vi "Get Min Meter ROI.vi"(8 "error in (no error)":errorcluster, 11 "Item Ref in":T2 format="%.0x") -> (0 "error out":errorcluster, 1 "empty?":bool, 2 "Max Gauge ROI":T1, 3 "Item Ref out":T2 format="%.0x")   [LabVIEW 2011, in "Meter Detection Custom Device.lvlib"]
uses:
  Meter Detection Custom Device.lvlib
  <vilib>/NI Veristand/Custom Device API/Custom Device Item Ref.ctl
  Meter Detection Global Variable.vi
  <vilib>/NI Veristand/Custom Device API/Get Item Property (Variant).vi
  <vilib>/NI Veristand/Custom Device API/Custom Device API.lvlib
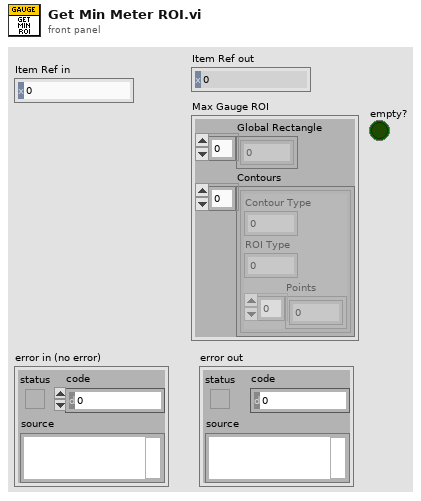
[diagram p1: front panel]
types:
  T1 = cluster{"Global Rectangle":i32[], "Contours":cluster{"Contour Type":u32, "ROI Type":u32, "Points":i32[]}[]}
  T2 = typedef "Custom Device API.lvlib/Custom Device Item Ref.ctl" = u64
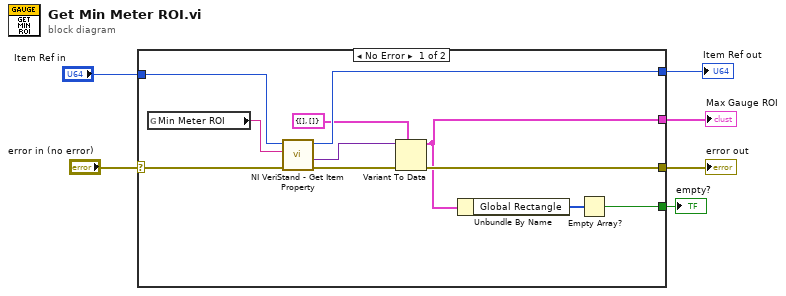
[diagram p0: block diagram]
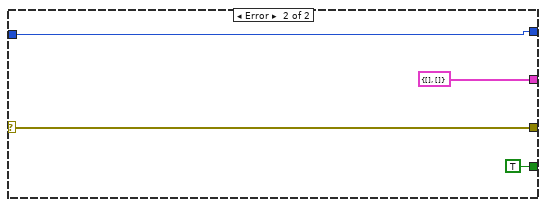
[diagram p2: hidden frame]
diagram:
  n1 = case shown="No Error" "error in (no error)" {
    selector: "error in (no error)" -> [w10 w21]
    tunnel: [w17 w20] -> w6
    tunnel: "Item Ref in" -> [w16 w20]
    tunnel: [w11 w21] -> w4
    tunnel: [w8 T1 {"Global Rectangle"=[], "Contours"=[]} ("ROI")] -> w3
    tunnel: [w7 TRUE ("empty?")] -> w1
    frame No Error {
      n2 = global read "Meter Detection Global Variable.vi" "Min Meter ROI"() -> (w15:string)
      n3 = call-poly <vilib>:"NI VeriStand - Get Item Property.vi"("error in (no error)"=w10, "Property Name"=w15, "Item Ref in"=w16) -> ("error out"=w13:errorcluster, "Value"=w12:variant, "Item Ref out"=w17:T2)  [unwired: 5 in, 1 out]
      n4 = Variant To Data(error in=w13, type=T1 {"Global Rectangle"=[], "Contours"=[]} ("ROI"), Variant=w12) -> (data=w8:T1, error out=w11:errorcluster)
      n5 = Unbundle By Name(w8) -> ("Global Rectangle"=w9:i32[])
      n6 = Empty Array?(array=w9) -> (empty?=w7:bool)
    }
    frame Error {
    }
  }
  "Item Ref out" <- w6
  "error out" <- w4
  "Max Gauge ROI" <- w3
  "empty?" <- w1
